vi "Fetch Double Variable Value.vi"(8 "error in (no error)":errorcluster, 10 "Variables":refnum<k24>[](array[refnum]), 11 "Identifier":string) -> (0 "error out":errorcluster, 2 "Variables dup":refnum<k24>[](array[refnum]), 3 "Value":dbl)   [LabVIEW 2011]
uses:
  NationalInstruments.VeriStand.RealTimeSequenceDefinitionApi
  NationalInstruments.VeriStand.DataTypes
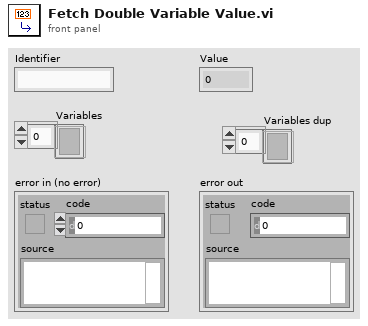
[diagram p1: front panel]
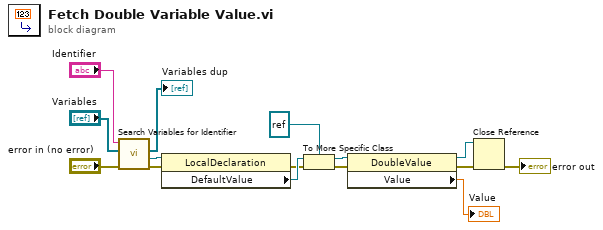
[diagram p0: block diagram]
diagram:
  n1 = call "Search Variables for Identifier.vi"("error in (no error)"="error in (no error)", "Variables"="Variables", "Identifier"="Identifier") -> ("error out"=w9:errorcluster, "Found Variable"=w4:refnum<k24>, "Variables dup"=→"Variables dup":refnum<k24>[])  [unwired: 6 in]
  n2 = property class="LocalDeclaration"(reference=w4, error in=w9) -> (error out=w10:errorcluster, "DefaultValue"=w11:refnum<k24>)  [unwired: 1 out]
  n3 = To More Specific Class(target class=refnum<k24> refnum, reference=w11, error in=w10) -> (specific class reference=w14:refnum<k24>, error out=w13:errorcluster)
  n4 = property class="DoubleValue"(reference=w14, error in=w13) -> (reference out=w2:refnum<k24>, error out=w3:errorcluster, "Value"=→"Value":dbl)
  n5 = Close Reference(reference=w2, error in (no error)=w3) -> (error out=→"error out":errorcluster)
